vi "Touch Panel Main.vi"() -> ()   [LabVIEW 2018]
doc: "使用该模板创建Touch Panel VI。"
panel:
  in  "选项卡控件":T1(tab)
  in  "换算<替换该项>":dbl(slide)=1.0 step=0.25 scale=0.0..10.0
  out "数据":dbl(graph)
  out "预警<替换该项>":bool
  in  "退出":bool
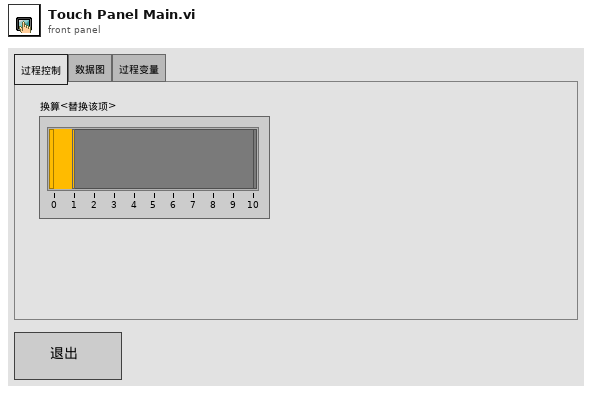
[diagram p1: front panel]
types:
  T1 = enum32{"Process Control", "Data Graph", "Process Variables"}
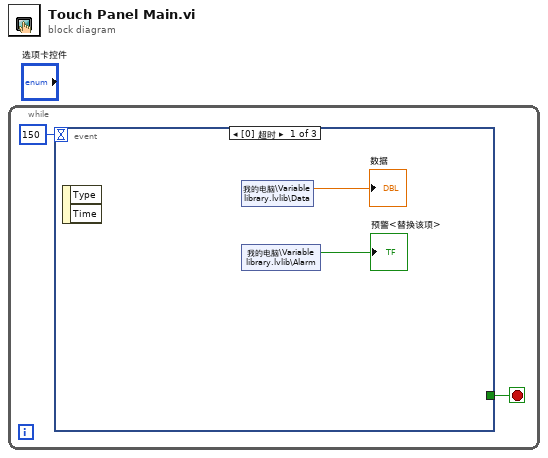
[diagram p0: block diagram]
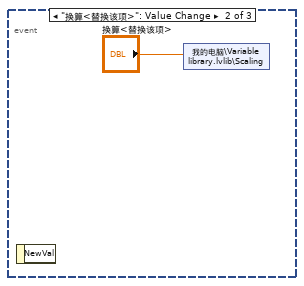
[diagram p2: hidden frame]
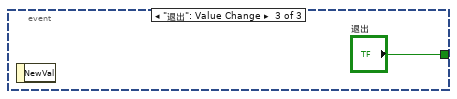
[diagram p3: hidden frame]
diagram:
  n1 = while {
    stop <- w2 stop-if-true
    n2 = event shown="[0] 超时" {
      selector: _ -> [_ _ _]
      dyn-events: _ -> [_ _ _]
      timeout: 150 -> [_ _ _]
      tunnel: [_ _ "退出"] -> w2
      event Timeout {
        n3 = event-data() -> ()  [unwired: 1 in, 2 out]
        n4 = shared-variable "我的电脑\\Variable library.lvlib\\Data"() -> (→"数据":dbl)  [unwired: 1 in, 1 out]
        n5 = shared-variable "我的电脑\\Variable library.lvlib\\Alarm"() -> (→"预警<替换该项>":bool)  [unwired: 1 in, 1 out]
      }
      event "换算<替换该项>": Value Change {
        n6 = event-data() -> ()  [unwired: 1 in, 1 out]
        n7 = shared-variable "我的电脑\\Variable library.lvlib\\Scaling"("换算<替换该项>") -> ()  [unwired: 1 in, 1 out]
      }
      event "退出": Value Change {
        n8 = event-data() -> ()  [unwired: 1 in, 1 out]
      }
    }
  }
